vi "ukol5.vi"() -> ()   [LabVIEW 2023]
uses:
  <vilib>/Analysis/2dsp.llb/Real FFT.vi
  <vilib>/Utility/file.llb/Read Delimited Spreadsheet (DBL).vi
  <vilib>/Analysis/NI_AALPro.lvlib
panel:
  out "Waveform Graph 2":waveform(dbl)[](graph)
  out "Waveform Graph":waveform(dbl)[](graph)
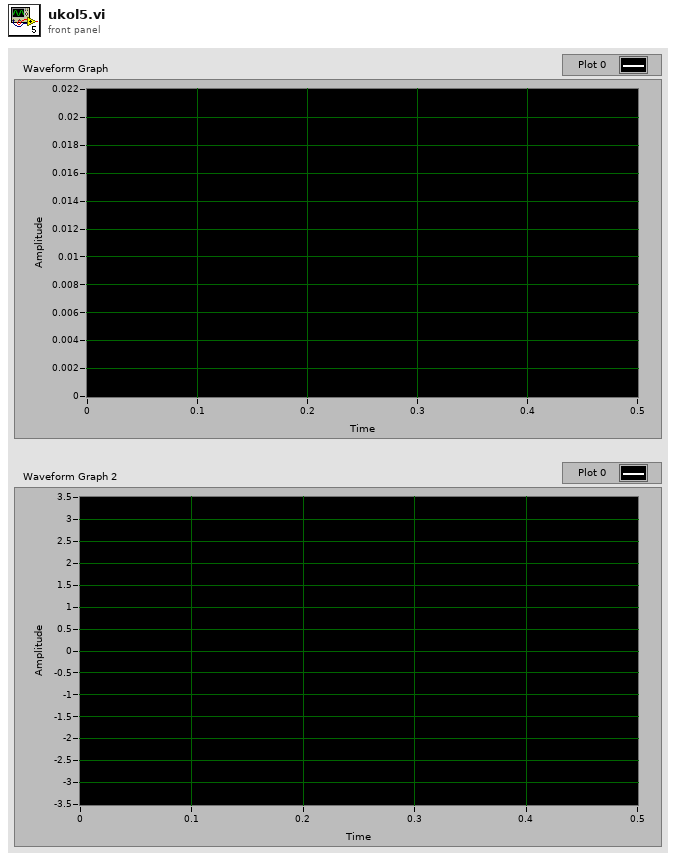
[diagram p1: front panel]
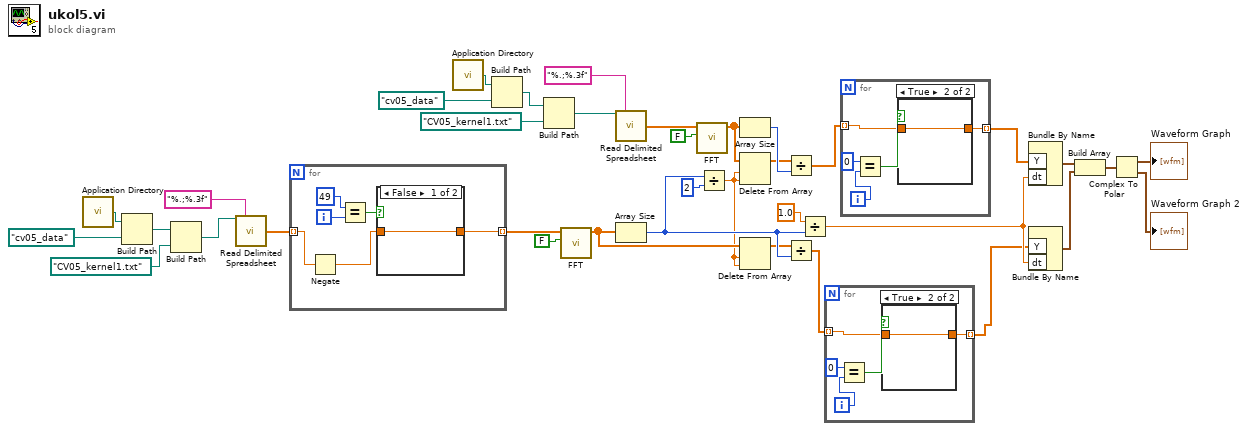
[diagram p0: block diagram]
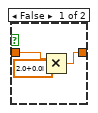
[diagram p2: hidden frame]
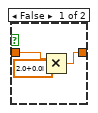
[diagram p3: hidden frame]
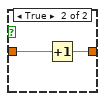
[diagram p4: hidden frame]
diagram:
  n1 = call <vilib>:"Application Directory.vi"() -> ("Application Directory"=w30:path)
  n2 = Build Path(base path=w30, name or relative path=path "cv05_data") -> (appended path=w28:path)
  n3 = Build Path(base path=w28, name or relative path=path "CV05_kernel1.txt") -> (appended path=w26:path)
  n4 = call-poly <vilib>:"Read Delimited Spreadsheet.vi"("file path (dialog if empty)"=w26, "format (%.3f)"="%.;%.3f") -> ("first row"=w24:dbl[])  [unwired: 8 in, 5 out]
  n5 = for {
    tunnel: w24 -> [w38] mode=indexing
    tunnel: [w39] -> w22 mode=indexing
    i -> [w42]
    n6 = Negate(x=w38) -> (-x=w37:dbl)
    n7 = Equal?(x=49, y=w42) -> (x = y?=w40:bool)
    n8 = case shown="False" w40 {
      tunnel: [w43 w45] -> w39
      tunnel: w37 -> [w43 w44]
      frame False {
      }
      frame True {
        n9 = Increment(x=w44) -> (x+1=w45:dbl)
      }
    }
  }
  n10 = call <vilib>:"Application Directory.vi"() -> ("Application Directory"=w36:path)
  n11 = Build Path(base path=w36, name or relative path=path "cv05_data") -> (appended path=w34:path)
  n12 = Build Path(base path=w34, name or relative path=path "CV05_kernel1.txt") -> (appended path=w32:path)
  n13 = call-poly <vilib>:"FFT.vi"("shift?"=FALSE, "X"=w22) -> ("FFT {X}"=w11:cdb[])  [unwired: 8 in, 1 out]
  n14 = call-poly <vilib>:"Read Delimited Spreadsheet.vi"("file path (dialog if empty)"=w32, "format (%.3f)"="%.;%.3f") -> ("first row"=w23:dbl[])  [unwired: 8 in, 5 out]
  n15 = Array Size(array=w11) -> (size(s)=w10:i32)
  n16 = call-poly <vilib>:"FFT.vi"("shift?"=FALSE, "X"=w23) -> ("FFT {X}"=w7:cdb[])  [unwired: 8 in, 1 out]
  n17 = Divide(x=w10, y=2) -> (x/y=w5:dbl)
  n18 = Array Size(array=w7) -> (size(s)=w21:i32)
  n19 = Delete From Array(array=w7, length=w5, index=w5) -> (array with subset deleted=w6:cdb[])  [unwired: 1 out]
  n20 = Delete From Array(array=w11, length=w5, index=w5) -> (array with subset deleted=w8:cdb[])  [unwired: 1 out]
  n21 = Divide(x=w6, y=w21) -> (x/y=w2:cdb[])
  n22 = Divide(x=w8, y=w10) -> (x/y=w4:cdb[])
  n23 = Divide(x=1.0, y=w10) -> (x/y=w14:dbl)
  n24 = for {
    tunnel: w4 -> [w46] mode=indexing
    tunnel: [w47] -> w3 mode=indexing
    i -> [w50]
    n25 = Equal?(x=0, y=w50) -> (x = y?=w48:bool)
    n26 = case shown="True" w48 {
      tunnel: [w51 w54] -> w47
      tunnel: w46 -> [w53 w54]
      frame False {
        n27 = Multiply(x=w53, y=cdb 2.0+0.0i) -> (x*y=w51:cdb)
      }
      frame True {
      }
    }
  }
  n28 = for {
    tunnel: w2 -> [w55] mode=indexing
    tunnel: [w56] -> w1 mode=indexing
    i -> [w59]
    n29 = Equal?(x=0, y=w59) -> (x = y?=w57:bool)
    n30 = case shown="True" w57 {
      tunnel: [w60 w63] -> w56
      tunnel: w55 -> [w62 w63]
      frame False {
        n31 = Multiply(x=w62, y=cdb 2.0+0.0i) -> (x*y=w60:cdb)
      }
      frame True {
      }
    }
  }
  n32 = Bundle By Name("Y"=w1, "dt"=w14) -> (w15:waveform(cdb))  [unwired: 1 in]
  n33 = Bundle By Name("Y"=w3, "dt"=w14) -> (w13:waveform(cdb))  [unwired: 1 in]
  n34 = Build Array(w15, w13) -> (w20:waveform(cdb)[])
  n35 = Complex To Polar(r * e^(i*theta)=w20) -> (r=→"Waveform Graph":waveform(dbl)[], theta=→"Waveform Graph 2":waveform(dbl)[])
